vi "ExposeGetVariantAttributeAsControl.vi"(10 "Name":string, 11 "Variant":variant) -> (1 "Found?":bool, 2 "Is Control?":bool, 3 "Ctl Ref":refnum<vi>)   [LabVIEW 2017]
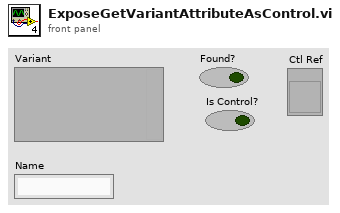
[diagram p1: front panel]
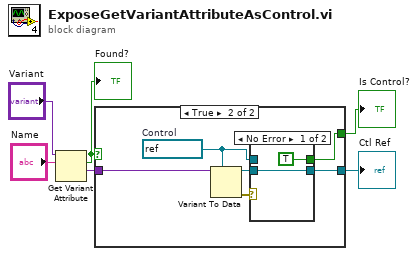
[diagram p0: block diagram]
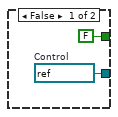
[diagram p2: hidden frame]
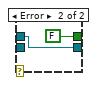
[diagram p3: hidden frame]
diagram:
  n1 = Get Variant Attribute(Variant="Variant", name="Name") -> (found=w6:bool, value=w5:variant)  [unwired: 2 in, 2 out]
  "Found?" <- w6
  n2 = case shown="True" w6 {
    tunnel: w5 -> [_ w14]
    tunnel: [w8 w11] -> w2
    tunnel: [FALSE w10] -> w1
    frame False {
      w8 = refnum<vi> refnum  # Control
    }
    frame True {
      w9 = refnum<vi> refnum  # Control
      n3 = Variant To Data(type=w9, Variant=w14) -> (data=w12:refnum<vi>, error out=w13:errorcluster)  [unwired: 1 in]
      n4 = case shown="No Error" w13 {
        tunnel: w12 -> [w16 _]
        tunnel: [w16 w17] -> w11
        tunnel: [TRUE FALSE] -> w10
        tunnel: w9 -> [_ w17]
        frame No Error {
        }
        frame Error {
        }
      }
    }
  }
  "Ctl Ref" <- w2
  "Is Control?" <- w1
